vi "Hantek Scope Tool.vi"() -> ()   [LabVIEW 2013]
uses:
  HTMarch.dll
panel:
  in  "DrawLen":u32=10000
  out "Scan Time (ms)":u32
  in  "ReadLen":i32=10240
  in  "stop":bool
  out "?":i16[][](graph)
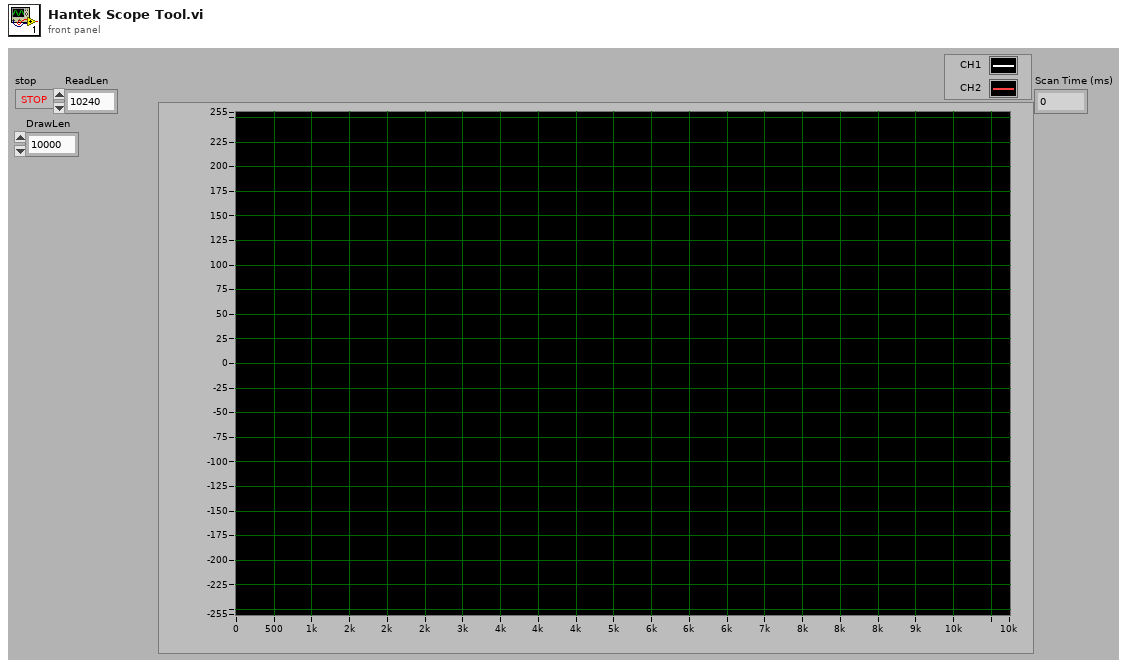
[diagram p1: front panel]
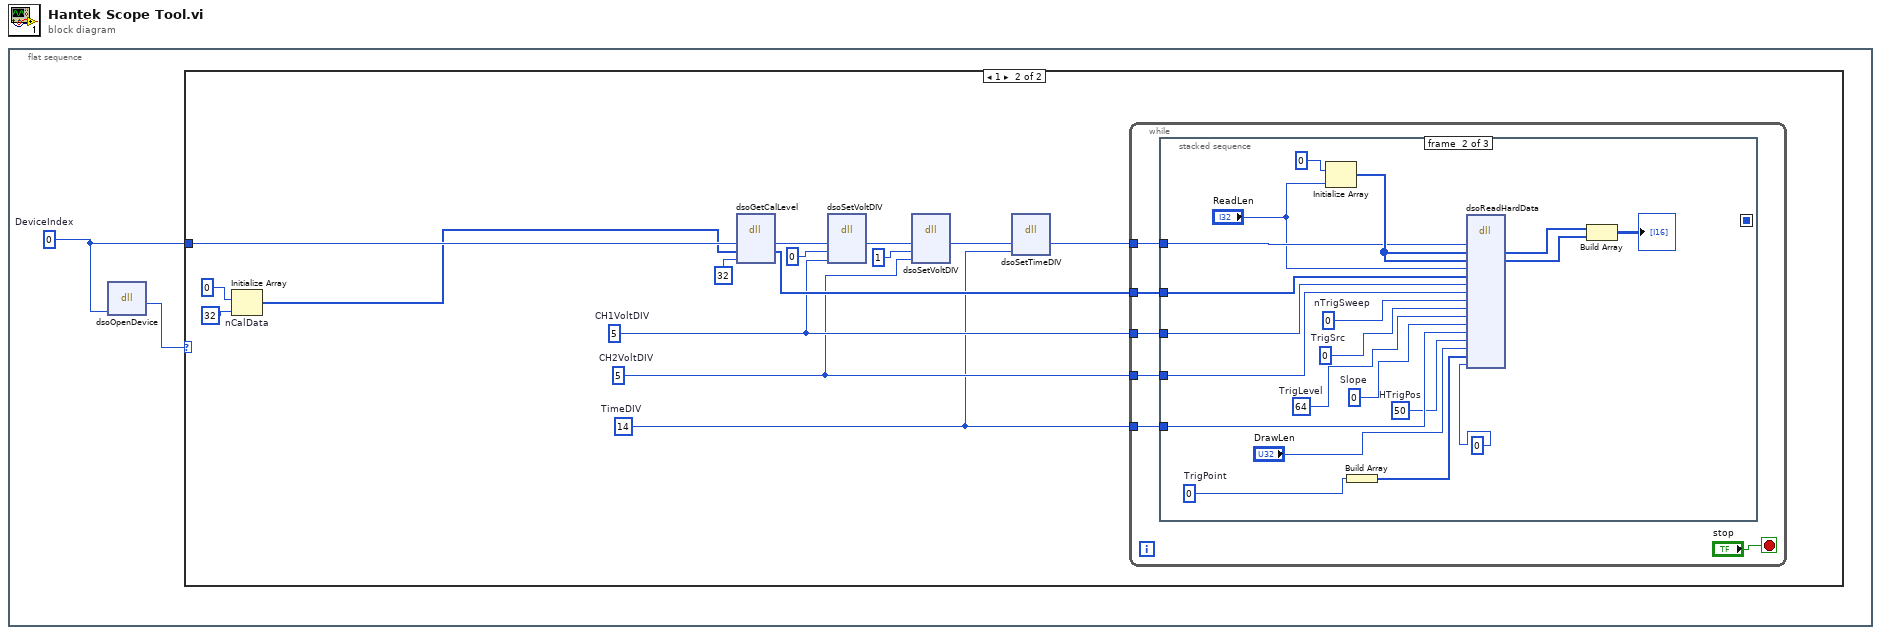
[diagram p0: block diagram]
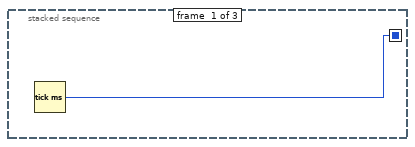
[diagram p3: hidden frame]
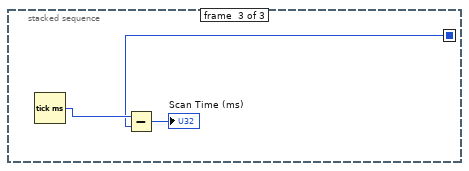
[diagram p4: hidden frame]
diagram:
  n1 = flat-sequence {
    frame #0 {
      w1 = u16 0  # DeviceIndex
      n2 = dll-call lib="E:/My Documents/GitHub/LabVIEW/Electronics/Hantek Oscilloscope/HTMarch.dll" fn="dsoOpenDevice" label="OpenDevice"("DeviceIndex"=w1) -> ("返回类型"=w2:i16)  [unwired: 4 in, 2 out]
      n3 = case shown="1" w2 {
        tunnel: w1 -> [_ w17]
        frame 0, Default {
        }
        frame 1 {
          w9 = 14  # TimeDIV
          w10 = 5  # CH2VoltDIV
          w11 = 5  # CH1VoltDIV
          n4 = Initialize Array "nCalData"(i16 0, 32) -> (w14:i16[])
          n5 = dll-call lib="E:/My Documents/GitHub/LabVIEW/Electronics/Hantek Oscilloscope/HTMarch.dll" fn="dsoGetCalLevel" label="GetCalLevel"("DeviceIndex"=w17, "level"=w14, "nLen"=i16 32) -> ("DeviceIndex"=w7:u16, "level"=w12:i16[])  [unwired: 5 in, 2 out]
          n6 = dll-call lib="E:/My Documents/GitHub/LabVIEW/Electronics/Hantek Oscilloscope/HTMarch.dll" fn="dsoSetVoltDIV" label="SetCh1VoltDIV"("DeviceIndex"=w7, "nCH"=0, "nVoltDIV"=w11) -> ("DeviceIndex"=w5:u16)  [unwired: 6 in, 2 out]
          n7 = dll-call lib="E:/My Documents/GitHub/LabVIEW/Electronics/Hantek Oscilloscope/HTMarch.dll" fn="dsoSetVoltDIV" label="SetCh2VoltDIV"("DeviceIndex"=w5, "nCH"=1, "nVoltDIV"=w10) -> ("DeviceIndex"=w3:u16)  [unwired: 6 in, 2 out]
          n8 = dll-call lib="E:/My Documents/GitHub/LabVIEW/Electronics/Hantek Oscilloscope/HTMarch.dll" fn="dsoSetTimeDIV" label="SetTimeDIV"("DeviceIndex"=w3, "nTimeBase"=w9) -> ("DeviceIndex"=w13:u16)  [unwired: 5 in, 2 out]
          n9 = while {
            tunnel: w13 -> [w23]
            tunnel: w12 -> [w22]
            tunnel: w11 -> [w21]
            tunnel: w10 -> [w20]
            tunnel: w9 -> [w19]
            stop <- "stop" stop-if-true
            n10 = stacked-sequence {
              seq-local: [w24 _ _] -> [_ _ w46]
              tunnel: w23 -> [_ w42 _]
              tunnel: w22 -> [_ w41 _]
              tunnel: w21 -> [_ w40 _]
              tunnel: w20 -> [_ w39 _]
              tunnel: w19 -> [_ w35 _]
              frame #0 {
                n11 = Tick Count (ms)() -> (millisecond timer value=w24:u32)
              }
              frame #1 {
                w29 = u32 0  # TrigPoint
                w33 = i16 50  # HTrigPos
                w34 = i16 0  # Slope
                w36 = i16 64  # TrigLevel
                w37 = i16 0  # TrigSrc
                w38 = i16 0  # nTrigSweep
                n12 = Initialize Array(i16 0, "ReadLen") -> (w43:i16[])
                n13 = Build Array(w29) -> (w28:u32[])
                n14 = dll-call lib="E:/My Documents/GitHub/LabVIEW/Electronics/Hantek Oscilloscope/HTMarch.dll" fn="dsoReadHardData" label="ReadHardData"("DeviceIndex"=w42, "pCH1Data"=w43, "pCH2Data"=w43, "nReadLen"="ReadLen", "pCalLevel"=w41, "nCH1VoltDIV"=w40, "nCH2VoltDIV"=w39, "nTrigSweep"=w38, "nTrigSrc"=w37, "nTrigLevel"=w36, "nSlope"=w34, "TimeDiv"=w35, "nHTrigPos"=w33, "nDisLen"="DrawLen", "nTrigPoint"=w28, "nInsertMode"=i16 0) -> ("pCH1Data"=w31:i16[], "pCH2Data"=w30:i16[])  [unwired: 18 in, 2 out]
                n15 = Build Array(w31, w30) -> (→"?":i16[][])
              }
              frame #2 {
                n16 = Tick Count (ms)() -> (millisecond timer value=w47:u32)
                n17 = Subtract(x=w47, y=w46) -> (x-y=→"Scan Time (ms)":u32)
              }
            }
          }
        }
      }
    }
  }
